vi "Read Module Name.vi"(8 "error in (no error)":errorcluster) -> (0 "error out":errorcluster, 3 "Module Name":string)   [LabVIEW 2015, in "Generic Module Library.lvlib" / "Template G_Module.lvlib"]
uses:
  Template G_Module.lvlib
  Module Class/Rename.lvclass
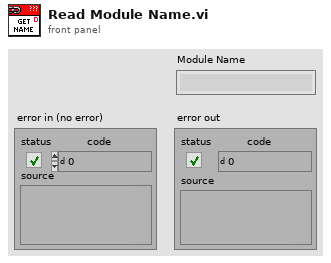
[diagram p1: front panel]
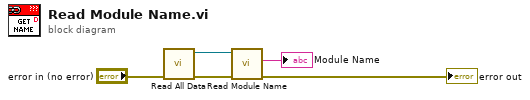
[diagram p0: block diagram]
diagram:
  n1 = call "Read All Data.vi"("error in (no error)"="error in (no error)") -> ("error out"=w3:errorcluster, "Data Out"=w4:refnum<class "Rename.lvclass">)  [unwired: 9 in]
  n2 = call-dynamic "Read Module Name.vi"("error in (no error)"=w3, "Rename in"=w4) -> ("error out"=→"error out":errorcluster, "Module Name"=→"Module Name":string)  [unwired: 7 in, 1 out]
